vi "SIFT align.vi"(6 "post image file":string="post.png", 7 "pre image file":string="pre.png", 8 "Inverse PNG":bool=TRUE, 9 "Affine":bool, 10 "smoothing radius":u16=2, 11 "working directory":path=path "D:/3D FIB-SEM Files") -> (0 "Delta image":dbl format="%#_3g", 1 "failed":bool, 2 "Delta Y":dbl format="%#_3g", 3 "Delta X":dbl format="%#_3g")   [LabVIEW 2018]
panel:
  out "Translation array":dbl[](array[numeric])
  out "Affine array":dbl[](array[numeric])
  out "SIFT.txt":string
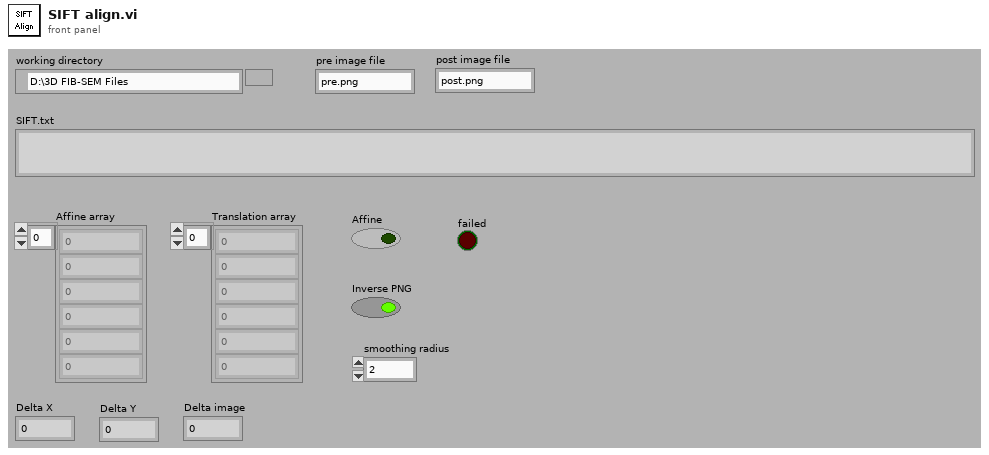
[diagram p1: front panel]
types:
  T1 = enum16{"open", "replace", "create", "open or create", "replace or create", "replace or create with confirmation"}
  T2 = typedef "imagedata.ctl" = cluster{"image type":i32, "image depth":i32, "image":u8[], "mask":u8[], "colors":u32[], "Rectangle":cluster{"left":i16, "top":i16, "right":i16, "bottom":i16}}
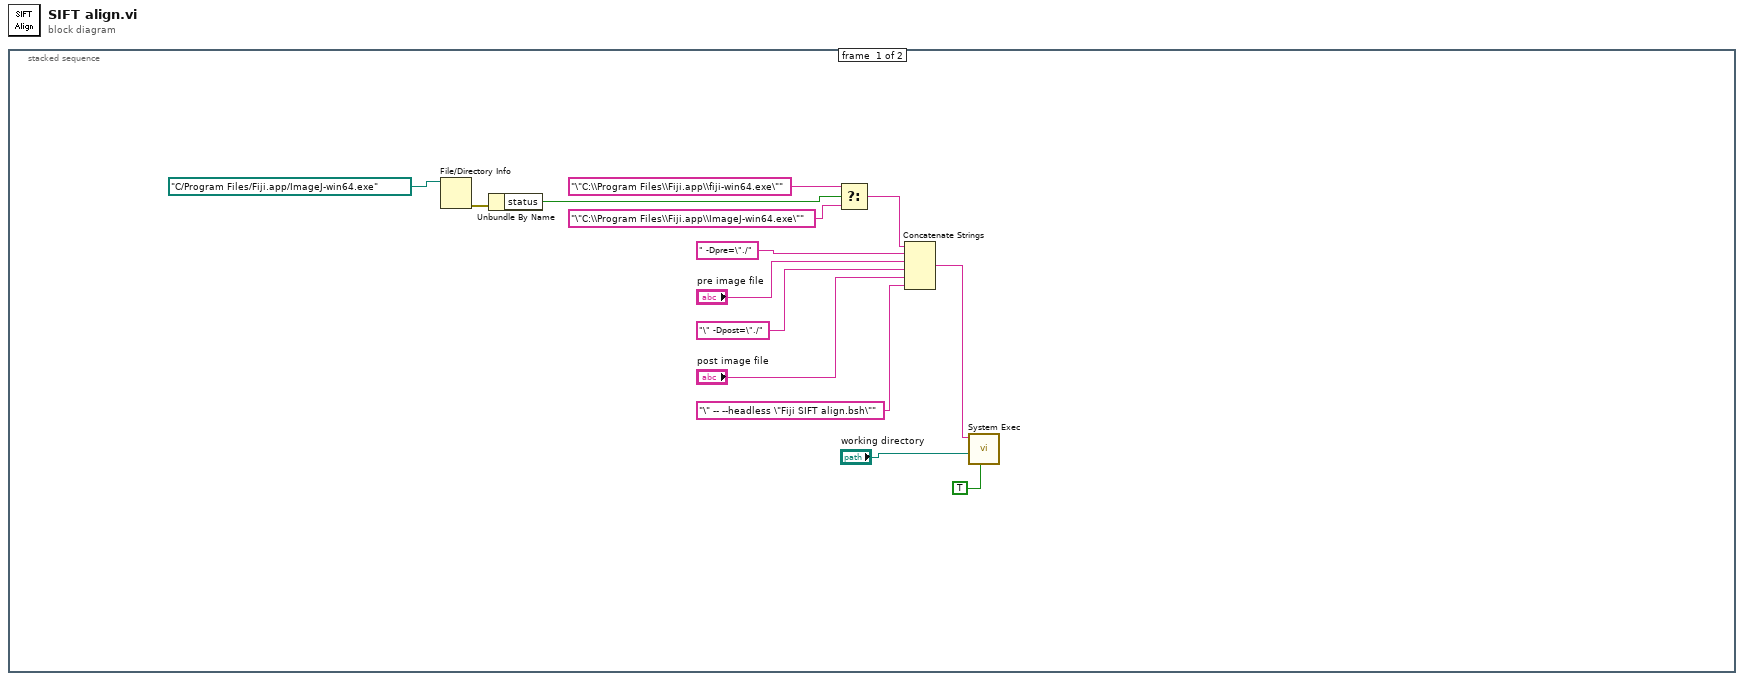
[diagram p0: block diagram]
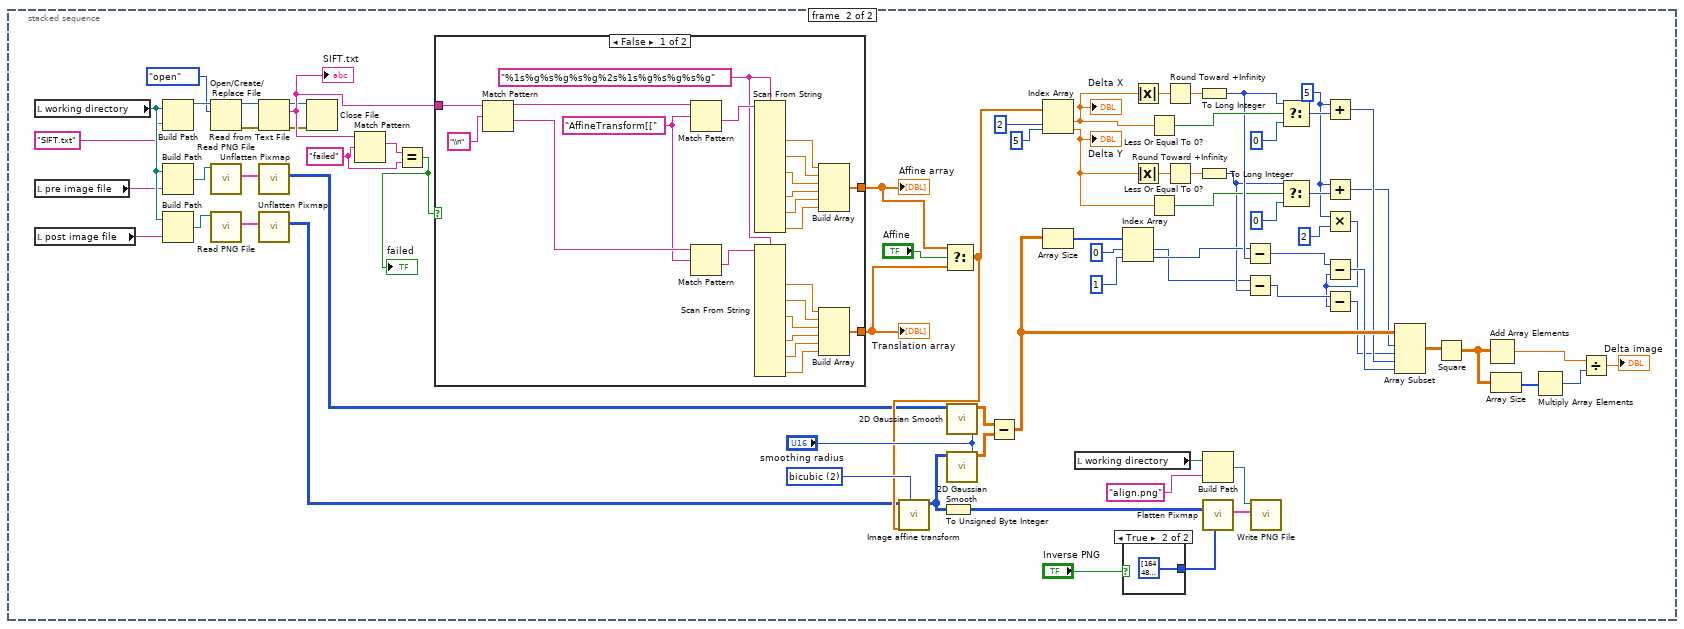
[diagram p2: hidden frame]
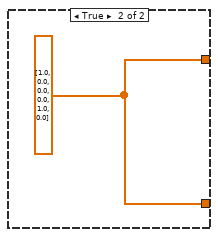
[diagram p3: hidden frame]
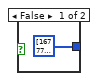
[diagram p4: hidden frame]
diagram:
  n1 = stacked-sequence {
    frame #0 {
      n2 = File/Directory Info(path=path "C:/Program Files/Fiji.app/ImageJ-win64.exe") -> (error out=w11:errorcluster)  [unwired: 1 in, 6 out]
      n3 = Unbundle By Name(w11) -> ("status"=w9:bool)
      n4 = Select(t="\"C:\\Program Files\\Fiji.app\\fiji-win64.exe\"" ("command line"), s=w9, f="\"C:\\Program Files\\Fiji.app\\ImageJ-win64.exe\"" ("command line")) -> (s? t:f=w7:string)
      n5 = Concatenate Strings(w7, " -Dpre=\"./" ("string"), "pre image file", "\" -Dpost=\"./" ("string"), "post image file", "\" -- --headless \"Fiji SIFT align.bsh\"" ("string")) -> (w6:string)
      n6 = call <vilib>:"System Exec.vi"("run minimized? (F)"=TRUE, "working directory"="working directory", "command line"=w6) -> ()  [unwired: 5 in, 4 out]
    }
    frame #1 {
      w20 = 5 ("x")
      w52 = "failed" ("regular expression")
      w74 = 2 items=["nearest", "bilinear", "bicubic", "bicubic spline"] ("method")
      n7 = local read "working directory"() -> (w80:path)
      n8 = local read "pre image file"() -> (w16:string)
      n9 = local read "post image file"() -> (w15:string)
      n10 = Build Path(base path=w80, name or relative path="SIFT.txt") -> (appended path=w87:path)
      n11 = Build Path(base path=w80, name or relative path=w16) -> (appended path=w79:path)
      n12 = Build Path(base path=w80, name or relative path=w15) -> (appended path=w81:path)
      n13 = Open/Create/Replace File(file path (use dialog)=w87, operation (0:open)=T1."open") -> (refnum out=w85:refnum<file>, error out=w84:errorcluster)  [unwired: 4 in, 1 out]
      n14 = call <vilib>:"Read PNG File.vi"("path to PNG file"=w79) -> ("image data"=w83:T2)  [unwired: 8 in, 2 out]
      n15 = call <vilib>:"Read PNG File.vi"("path to PNG file"=w81) -> ("image data"=w82:T2)  [unwired: 8 in, 2 out]
      n16 = Read from Text File(file (use dialog)=w85, error in=w84) -> (refnum out=w47:refnum<file>, text=w54:string, error out=w48:errorcluster)  [unwired: 2 in, 1 out]
      "SIFT.txt" <- w54
      n17 = call <vilib>:"Unflatten Pixmap.vi"("image data"=w83) -> ("8-bit pixmap"=w50:u8[][])  [unwired: 4 in, 6 out]
      n18 = call <vilib>:"Unflatten Pixmap.vi"("image data"=w82) -> ("8-bit pixmap"=w49:u8[][])  [unwired: 4 in, 6 out]
      n19 = Close File(refnum=w47, error in=w48) -> ()  [unwired: 2 out]
      n20 = Match Pattern(string=w54, regular expression=w52) -> (match substring=w53:string)  [unwired: 1 in, 3 out]
      n21 = Equal?(x=w53, y=w52) -> (x = y?=w51:bool)
      "failed" <- w51
      n22 = case shown="False" w51 {
        tunnel: [w90 w110] -> w62
        tunnel: [w89 w110] -> w61
        tunnel: w54 -> [w88 _]
        frame False {
          w91 = "%1s%g%s%g%s%g%2s%1s%g%s%g%s%g" ("format string")
          w92 = "AffineTransform[[" ("regular expression")
          n23 = Match Pattern(string=w88, regular expression="\\n") -> (before substring=w108:string, after substring=w93:string)  [unwired: 1 in, 2 out]
          n24 = Match Pattern(string=w108, regular expression=w92) -> (after substring=w107:string)  [unwired: 1 in, 3 out]
          n25 = Match Pattern(string=w93, regular expression=w92) -> (after substring=w94:string)  [unwired: 1 in, 3 out]
          n26 = Scan From String(format string=w91, input string=w107) -> (output 2=w106:dbl, output 4=w105:dbl, output 6=w104:dbl, output 9=w103:dbl, output 11=w102:dbl, output 13=w101:dbl)  [unwired: 22 in, 3 out]
          n27 = Scan From String(format string=w91, input string=w94) -> (output 2=w95:dbl, output 4=w96:dbl, output 6=w97:dbl, output 9=w98:dbl, output 11=w99:dbl, output 13=w100:dbl)  [unwired: 22 in, 3 out]
          n28 = Build Array(w106, w105, w104, w103, w102, w101) -> (w90:dbl[])
          n29 = Build Array(w95, w96, w97, w98, w99, w100) -> (w89:dbl[])
        }
        frame True {
          w110 = dbl[] [1.0, 0.0, 0.0, 0.0, 1.0, 0.0]
        }
      }
      "Affine array" <- w62
      "Translation array" <- w61
      n30 = Select(t=w62, s="Affine", f=w61) -> (s? t:f=w59:dbl[])
      n31 = call "Image affine transform.vi"("method"=w74, "Affine array"=w59, "Input image"=w49) -> ("Output image"=w67:i16[][])  [unwired: 8 in]
      n32 = To Unsigned Byte Integer(number=w67) -> (unsigned 8bit integer=w69:u8[][])
      n33 = call "2D Gaussian Smooth.vi"("radius"="smoothing radius", "Input"=w50) -> ("Output"=w65:dbl[][])  [unwired: 8 in, 1 out]
      n34 = call "2D Gaussian Smooth.vi"("radius"="smoothing radius", "Input"=w67) -> ("Output"=w66:dbl[][])  [unwired: 8 in, 1 out]
      n35 = Subtract(x=w65, y=w66) -> (x-y=w46:dbl[][])
      n36 = Index Array(array=w59, index #1=2 ("index"), index #2=5 ("index")) -> (element #1=w42:dbl, element #2=w31:dbl)
      "Delta X" <- w42
      "Delta Y" <- w31
      n37 = Array Size(array=w46) -> (size(s)=w45:i32[])
      n38 = local read "working directory"() -> (w76:path)
      n39 = Index Array(array=w45, index #1=0 ("index"), index #2=1 ("index")) -> (element #1=w29:i32, element #2=w36:i32)
      n40 = case shown="True" "Inverse PNG" {
        tunnel: [u32[] [16777222, 65793, 131586, 197379, 263172, 328965, 394758, 460551, 526344, 592137, 657930, 723723, 789516, 855309, 921102, 986895, 1052688, 1118481, 1184274, 1250067, 1315860, 1381653, 1447446, 1513239, 1579032, 1644825, 1710618, 1776411, 1842204, 1907997, 1973790, 2039583, 2105376, 2171169, 2236962, 2302755, 2368548, 2434341, 2500134, 2565927, 2631720, 2697513, 2763306, 2829099, 2894892, 2960685, 3026478, 3092271, 3158064, 3223857, 3289650, 3355443, 3421236, 3487029, 3552822, 3618615, 3684408, 3750201, 3815994, 3881787, 3947580, 4013373, 4079166, 4144959, 4210752, 4276545, 4342338, 4408131, 4473924, 4539717, 4605510, 4671303, 4737096, 4802889, 4868682, 4934475, 5000268, 5066061, 5131854, 5197647, 5263440, 5329233, 5395026, 5460819, 5526612, 5592405, 5658198, 5723991, 5789784, 5855577, 5921370, 5987163, 6052956, 6118749, 6184542, 6250335, 6316128, 6381921, 6447714, 6513507, 6579300, 6645093, 6710886, 6776679, 6842472, 6908265, 6974058, 7039851, 7105644, 7171437, 7237230, 7303023, 7368816, 7434609, 7500402, 7566195, 7631988, 7697781, 7763574, 7829367, 7895160, 7960953, 8026746, 8092539, 8158332, 8224125, 8289918, 8355711, 8421504, 8487297, 8553090, 8618883, 8684676, 8750469, 8816262, 8882055, 8947848, 9013641, 9079434, 9145227, 9211020, 9276813, 9342606, 9408399, 9474192, 9539985, 9605778, 9671571, 9737364, 9803157, 9868950, 9934743, 10000536, 10066329, 10132122, 10197915, 10263708, 10329501, 10395294, 10461087, 10526880, 10592673, 10658466, 10724259, 10790052, 10855845, 10921638, 10987431, 11053224, 11119017, 11184810, 11250603, 11316396, 11382189, 11447982, 11513775, 11579568, 11645361, 11711154, 11776947, 11842740, 11908533, 11974326, 12040119, 12105912, 12171705, 12237498, 12303291, 12369084, 12434877, 12500670, 12566463, 12632256, 12698049, 12763842, 12829635, 12895428, 12961221, 13027014, 13092807, 13158600, 13224393, 13290186, 13355979, 13421772, 13487565, 13553358, 13619151, 13684944, 13750737, 13816530, 13882323, 13948116, 14013909, 14079702, 14145495, 14211288, 14277081, 14342874, 14408667, 14474460, 14540253, 14606046, 14671839, 14737632, 14803425, 14869218, 14935011, 15000804, 15066597, 15132390, 15198183, 15263976, 15329769, 15395562, 15461355, 15527148, 15592941, 15658734, 15724527, 15790320, 15856113, 15921906, 15987699, 16053492, 16119285, 16185078, 16250871, 16316664, 16382457, 16448250, 16514043, 16579836, 16645629, 16711422, 16448250] ("256 gray scale") u32[] [16448250, 16711422, 16645629, 16579836, 16514043, 16448250, 16382457, 16316664, 16250871, 16185078, 16119285, 16053492, 15987699, 15921906, 15856113, 15790320, 15724527, 15658734, 15592941, 15527148, 15461355, 15395562, 15329769, 15263976, 15198183, 15132390, 15066597, 15000804, 14935011, 14869218, 14803425, 14737632, 14671839, 14606046, 14540253, 14474460, 14408667, 14342874, 14277081, 14211288, 14145495, 14079702, 14013909, 13948116, 13882323, 13816530, 13750737, 13684944, 13619151, 13553358, 13487565, 13421772, 13355979, 13290186, 13224393, 13158600, 13092807, 13027014, 12961221, 12895428, 12829635, 12763842, 12698049, 12632256, 12566463, 12500670, 12434877, 12369084, 12303291, 12237498, 12171705, 12105912, 12040119, 11974326, 11908533, 11842740, 11776947, 11711154, 11645361, 11579568, 11513775, 11447982, 11382189, 11316396, 11250603, 11184810, 11119017, 11053224, 10987431, 10921638, 10855845, 10790052, 10724259, 10658466, 10592673, 10526880, 10461087, 10395294, 10329501, 10263708, 10197915, 10132122, 10066329, 10000536, 9934743, 9868950, 9803157, 9737364, 9671571, 9605778, 9539985, 9474192, 9408399, 9342606, 9276813, 9211020, 9145227, 9079434, 9013641, 8947848, 8882055, 8816262, 8750469, 8684676, 8618883, 8553090, 8487297, 8421504, 8355711, 8289918, 8224125, 8158332, 8092539, 8026746, 7960953, 7895160, 7829367, 7763574, 7697781, 7631988, 7566195, 7500402, 7434609, 7368816, 7303023, 7237230, 7171437, 7105644, 7039851, 6974058, 6908265, 6842472, 6776679, 6710886, 6645093, 6579300, 6513507, 6447714, 6381921, 6316128, 6250335, 6184542, 6118749, 6052956, 5987163, 5921370, 5855577, 5789784, 5723991, 5658198, 5592405, 5526612, 5460819, 5395026, 5329233, 5263440, 5197647, 5131854, 5066061, 5000268, 4934475, 4868682, 4802889, 4737096, 4671303, 4605510, 4539717, 4473924, 4408131, 4342338, 4276545, 4210752, 4144959, 4079166, 4013373, 3947580, 3881787, 3815994, 3750201, 3684408, 3618615, 3552822, 3487029, 3421236, 3355443, 3289650, 3223857, 3158064, 3092271, 3026478, 2960685, 2894892, 2829099, 2763306, 2697513, 2631720, 2565927, 2500134, 2434341, 2368548, 2302755, 2236962, 2171169, 2105376, 2039583, 1973790, 1907997, 1842204, 1776411, 1710618, 1644825, 1579032, 1513239, 1447446, 1381653, 1315860, 1250067, 1184274, 1118481, 1052688, 986895, 921102, 855309, 789516, 723723, 657930, 592137, 526344, 460551, 394758, 328965, 263172, 197379, 131586, 65793, 16777222] ("256 gray scale inverse")] -> w56
        frame False {
        }
        frame True {
        }
      }
      n41 = Absolute Value(x=w42) -> (abs(x)=w41:dbl)
      n42 = Absolute Value(x=w31) -> (abs(x)=w32:dbl)
      n43 = Less Or Equal To 0?(x=w42) -> (x <= 0?=w39:bool)
      n44 = Less Or Equal To 0?(x=w31) -> (x <= 0?=w34:bool)
      n45 = Round Toward +Infinity(x=w41) -> (ceil(x): smallest int >= x=w40:dbl)
      n46 = Round Toward +Infinity(x=w32) -> (ceil(x): smallest int >= x=w33:dbl)
      n47 = To Long Integer(number=w40) -> (32bit integer=w37:i32)
      n48 = To Long Integer(number=w33) -> (32bit integer=w30:i32)
      n49 = Build Path(base path=w76, name or relative path="align.png") -> (appended path=w75:path)
      n50 = call <vilib>:"Flatten Pixmap.vi"("colors"=w56, "8-bit pixmap"=w69) -> ("image data"=w78:T2)  [unwired: 4 in, 5 out]
      n51 = Subtract(x=w36, y=w37) -> (x-y=w24:i32)
      n52 = Subtract(x=w29, y=w30) -> (x-y=w22:i32)
      n53 = call <vilib>:"Write PNG File.vi"("image data"=w78, "path to PNG file"=w75) -> ()  [unwired: 8 in, 2 out]
      n54 = Select(t=w37, s=w39, f=0 ("element")) -> (s? t:f=w28:i32)
      n55 = Select(t=w30, s=w34, f=0 ("element")) -> (s? t:f=w25:i32)
      n56 = Add(x=w20, y=w28) -> (x+y=w27:i32)
      n57 = Add(x=w20, y=w25) -> (x+y=w26:i32)
      n58 = Multiply(x=w20, y=2) -> (x*y=w18:i32)
      n59 = Subtract(x=w24, y=w18) -> (x-y=w23:i32)
      n60 = Subtract(x=w22, y=w18) -> (x-y=w21:i32)
      n61 = Array Subset(array=w46, index (row)=w26, length (row)=w21, index (col)=w27, length (col)=w23) -> (w73:dbl[][])
      n62 = Square(x=w73) -> (x^2=w68:dbl[][])
      n63 = Add Array Elements(numeric array=w68) -> (sum=w71:dbl)
      n64 = Array Size(array=w68) -> (size(s)=w72:i32[])
      n65 = Multiply Array Elements(1:w72) -> (0:w70:i32)
      n66 = Divide(x=w71, y=w70) -> (x/y=→"Delta image":dbl)
    }
  }
